vi "Read JSON Config.vi"(8 "error in (no error)":errorcluster, 10 "JSON Config":string, 11 "Abs_Type in":refnum<class "Abs_Type.lvclass">) -> (0 "error out":errorcluster, 3 "Abs_Type out":refnum<class "Abs_Type.lvclass">)   [LabVIEW 2021, in "Abs_Type.lvclass"]
uses:
  Abs_Type.lvclass
  Abs_Type.lvclass/Abs_Type.ctl
  5a3659ea-1f73-454d-a190-80946acc92b4.vi
  <vilib>/JDP Science/JSONtext/Find Item.vi
  <vilib>/JDP Science/JSONtext/Next JSON Value.vi
  <vilib>/JDP Science/JSONtext/String Subset.vi
  <vilib>/JDP Science/JSONtext/Parsing/Advance past next JSON Value (inlined COPY).vi
  <vilib>/JDP Science/JSONtext/Parsing/Advance past whitespace.vi
  <vilib>/JDP Science/JSONtext/Parsing/Advance past String.vi
  <vilib>/JDP Science/JSONtext/Parsing/Advance past Number.vi
  <vilib>/JDP Science/JSONtext/Parsing/Advance past Line Ending.vi
  <vilib>/Utility/LVClass/Get LV Class Name.vi
  <vilib>/JDP Science/JSONtext/Parsing/Parse Full Path or Item Name.vi
  <vilib>/JDP Science/JSONtext/Parsing/Advance past Array.vi
  <vilib>/JDP Science/JSONtext/Parsing/Advance past Object.vi
  <vilib>/JDP Science/JSONtext/support/Error Cluster From Code.vi
  <vilib>/JDP Science/JSONtext/Offset/Find Item Locations by Path.vi
  <vilib>/JDP Science/JSONtext/JSON text to Variant.vi
  <vilib>/JDP Science/JSONtext/LVClass Serializer/JSONtext LVClass Serializer.lvclass
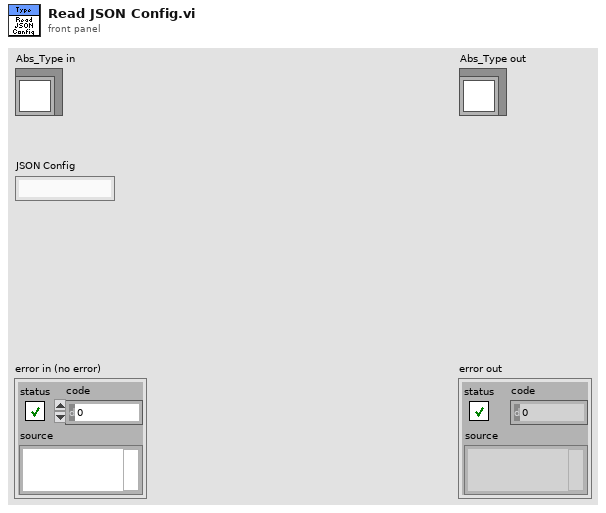
[diagram p1: front panel]
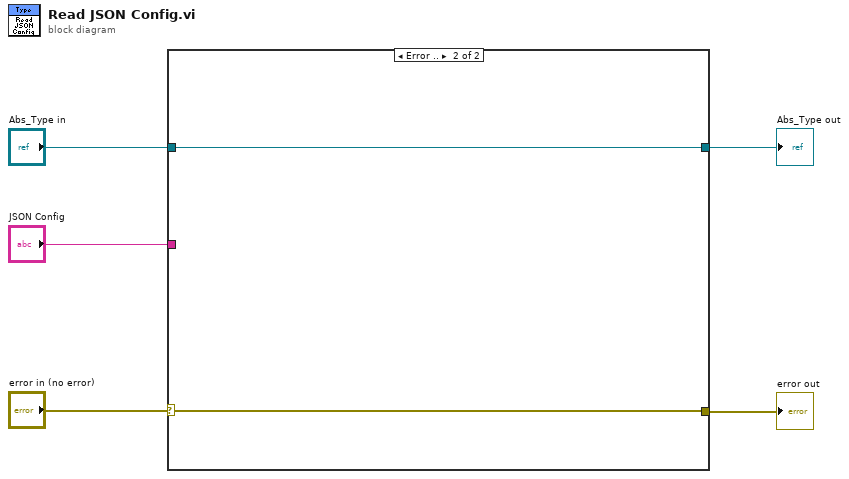
[diagram p0: block diagram]
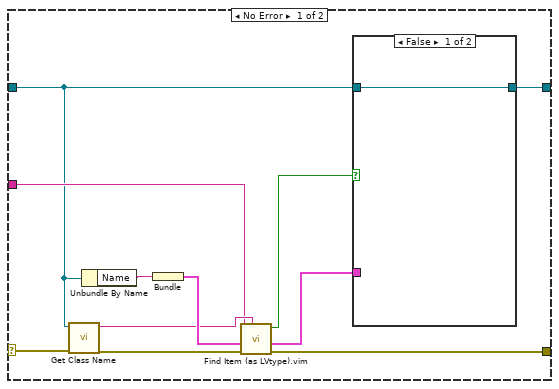
[diagram p2: hidden frame]
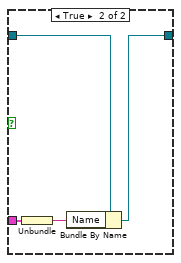
[diagram p3: hidden frame]
diagram:
  n1 = case shown="Error .." "error in (no error)" {
    selector: "error in (no error)" -> [w16 w22]
    tunnel: "JSON Config" -> [w12 _]
    tunnel: "Abs_Type in" -> [w9 w23]
    tunnel: [w8 w23] -> w2
    tunnel: [w7 w22] -> w1
    frame No Error {
      n2 = call "Get Class Name.vi"("error in (no error)"=w16, "Abs_Type in"=w9) -> ("error out"=w11:errorcluster, "class name"=w13:string)  [unwired: 8 in]
      n3 = Unbundle By Name(w9) -> ("Name"=w15:string)
      n4 = Bundle("Name"=w15) -> (w14:cluster{"Name":string})  [unwired: 1 in]
      n5 = call "Find Item (as LVtype).vim"("$Path or Item Name"=w13, "error in (no error)"=w11, "Data Type and Default Value"=w14, "JSON"=w12) -> ("error out"=w7:errorcluster, "Data"=w10:cluster{"Name":string}, "Found"=w6:bool)  [unwired: 4 in, 1 out]
      n6 = case shown="False" w6 {
        tunnel: w10 -> [_ w21]
        tunnel: w9 -> [w17 w20]
        tunnel: [w17 w18] -> w8
        frame False {
        }
        frame True {
          n7 = Unbundle(w21) -> ("Name"=w19:string)
          n8 = Bundle By Name(cluster=w20, "Name"=w19) -> (w18:refnum<class "Abs_Type.lvclass">)
        }
      }
    }
    frame Error {
    }
  }
  "error out" <- w1
  "Abs_Type out" <- w2
